vi "Test2_3a_ASIC_mezzanine.vi"(4 "Voltages comprobation":dbl[](array[numeric])=[0.05, 0.1, 0.2, 0.3, 0.4, 0.5, 0.6, 0.7, 0.8, 1.0], 6 "IB_Clip":i32[](array[numeric])=[0, 1, 2, 3, 4, 5, 6], 7 "Report Enable":bool, 8 "error in":errorcluster, 9 "Cycles Burst":i32=10000, 10 "Channels":i32[](array[numeric])=[0, 1, 2, 3, 4, 5, 6], 11 "Instrument VISA in":T1={"AWG VISA"="generadorpulsos", "Oscilloscope  VISA "="Oscilloscope", "Integration Board IP"="172.16.7.43", "connection ID"=refnum, "report out"=refnum, "report file path"=path "D:/CTA/Data_test/ASIC/chip_test"}) -> (0 "error out":errorcluster, 3 "Instrument VISA out":T1={"AWG VISA"="generadorpulsos", "Oscilloscope  VISA "="Oscilloscope", "Integration Board IP"="172.16.7.43", "connection ID"=refnum, "report out"=refnum, "report file path"=path "D:/CTA/Data_test/test3a"})   [LabVIEW 2009]
uses:
  <vilib>/Utility/NIReport.llb/NI_report.lvclass
  <vilib>/Utility/NIReport.llb/HTML/NI_HTML.lvclass
  <instrlib>/Agilent 8000 Series/Public/Configure/Configure Math (Binary Operation).vi
  <instrlib>/Agilent 8000 Series/Public/Data/Read (Multiple Waveforms).vi
  L0 Asic Test Folder v9/C/Program Files/National Instruments/LabVIEW 2012/instr.lib/Agilent 81150/Agilent 81150.lvlib
  L0 Asic Test Folder v9/C/Program Files/National Instruments/LabVIEW 2012/instr.lib/Agilent 8000 Series/Agilent 8000 Series.lvlib
panel:
  in  "Atenuation":i32[](array[numeric])=[0, 4, 8, 12]
  in  "Generador enable?":bool=TRUE
  out "dt":dbl
  out "report file path":path=path "D:/CTA/Data_test/ASIC/chip_test"
  in  "Full waveform":bool
  out "Waveform Data":waveform(dbl)[](graph)
  out "x-y 4":u32=42918
  in  "y":dbl=250.0
  out "bucle":u16
  out "x-y 3":u32=42918
  out "points quantity":dbl=104.0
  out "appended array":dbl[](array[numeric])=[1.222, 0.0079, 2.4586e-09, 6.8e-12, 0.009395, 0.004623, 9.99999e+37, 9.99999e+37, 5.8615e-09, 1.47682e-09, 104.0]
  out "read buffer 3":string="V amptd(1),1.233E+00,0,1.206E+00,1.250E+00,1.2220E+00,7.9E-03,1.04E+02,+ width(f1),2.471E-09,1,2.449E-09,2.472E-09,2.4586E-09,6.8E-12,1.03E+02,V amptd(f2),8.62E-03,1,1.99E-03,3.271E-02,9.395E-03,4.623E-03,1.04E+02,+ width(f2),9.99999E+37,5,9.99999E+37,9.99999E+37,9.99999E+37,9.99999E+37,9.99999E+37,Time(f1-f2),9.99999E+37,5,4.91554E-09,8.06319E-09,5.86150E-09,1.47682E-09,4E+00\n"
  out "x-y":u32=956
  out "Numeric":i32=2147483647
  in  "Att gain":u32=4095
  in  "Save NOW!":bool
  in  "End 2":bool=TRUE
  out "Data output":dbl[][](array[numeric])
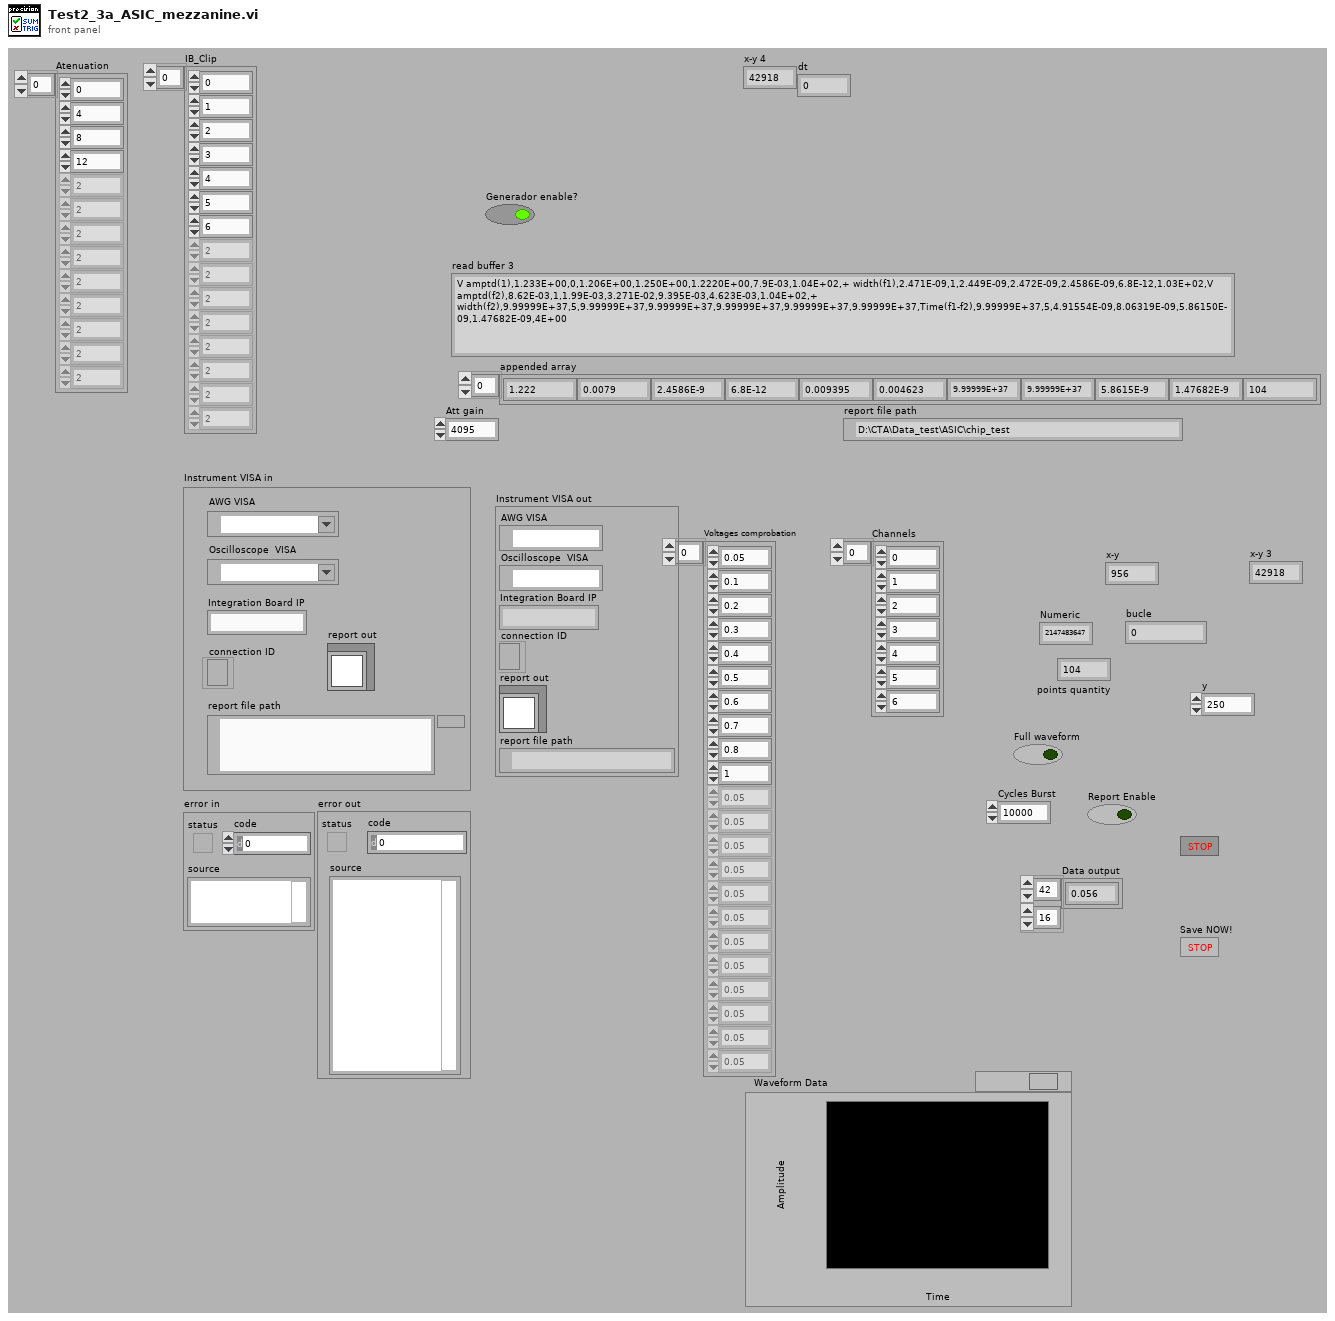
[diagram p1: front panel]
types:
  T1 = cluster{"AWG VISA":refnum<visa-resource-name>, "Oscilloscope  VISA ":refnum<visa-resource-name>, "Integration Board IP":string, "connection ID":refnum<k5>, "report out":refnum<class "NI_report.lvclass">, "report file path":path}
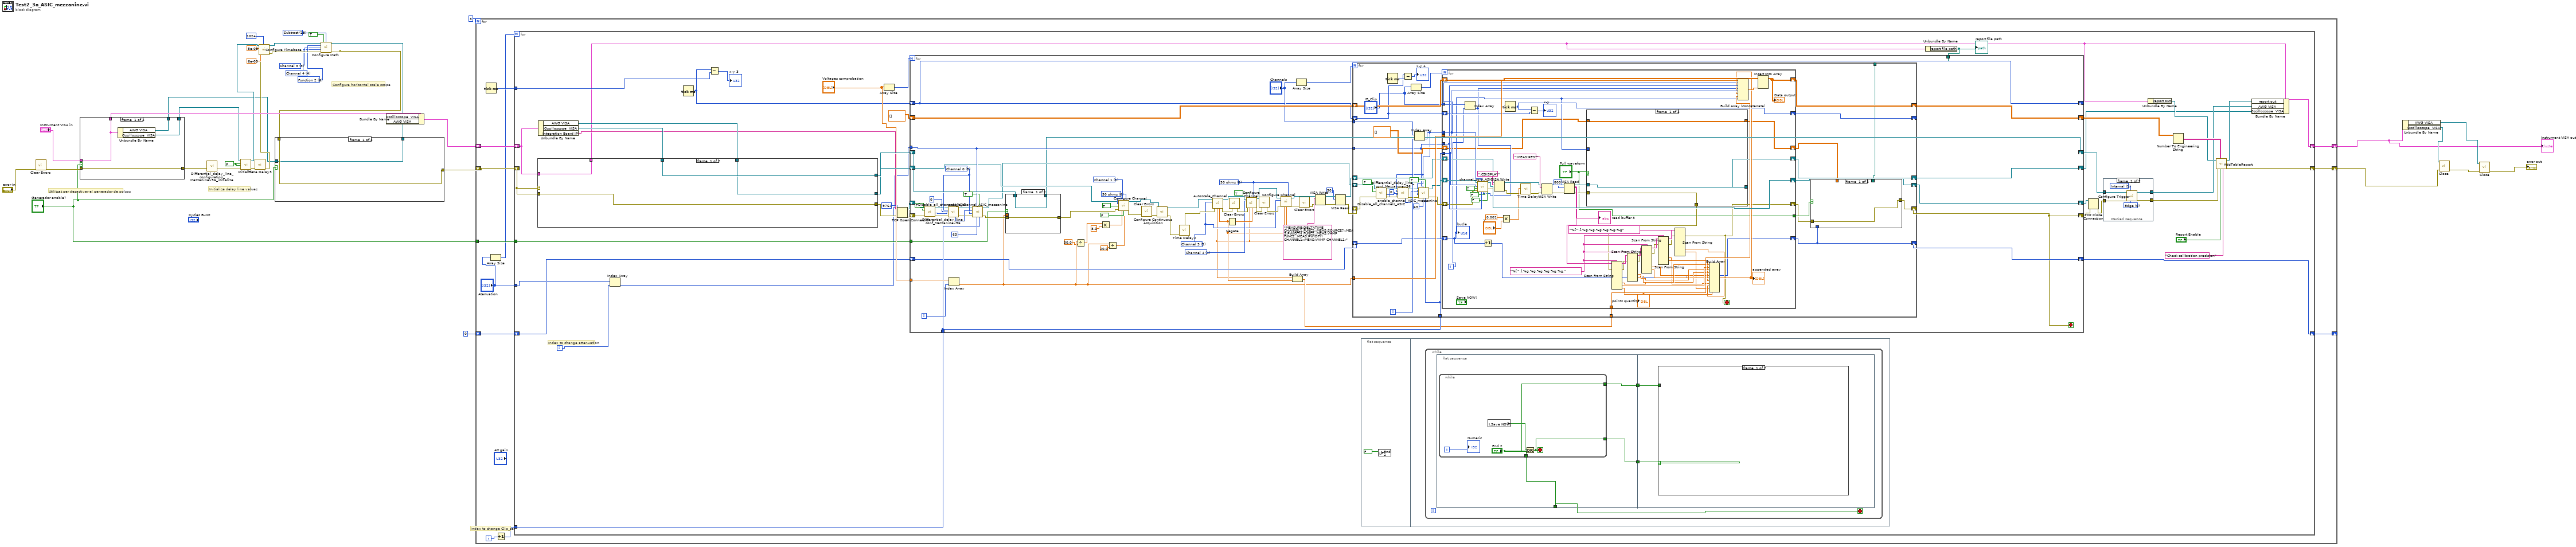
[diagram p0: block diagram]
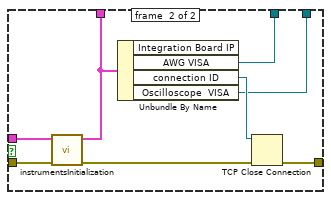
[diagram p2: hidden frame]
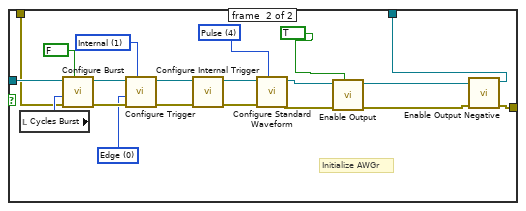
[diagram p3: hidden frame]
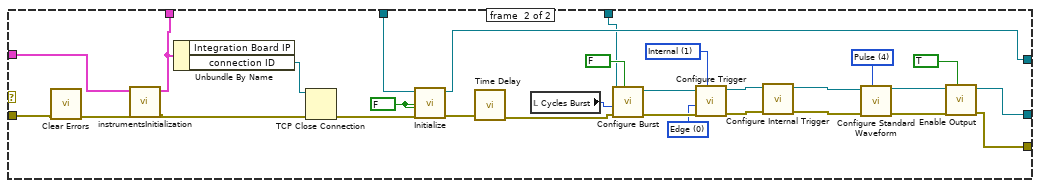
[diagram p4: hidden frame]
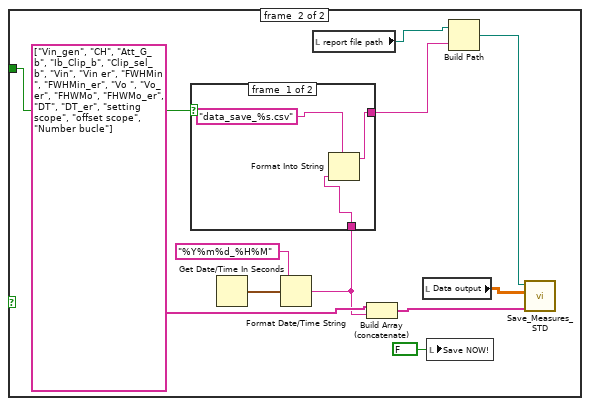
[diagram p5: hidden frame]
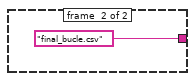
[diagram p6: hidden frame]
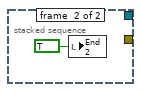
[diagram p7: hidden frame]
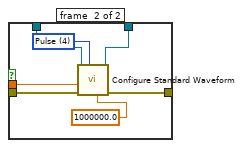
[diagram p8: hidden frame]
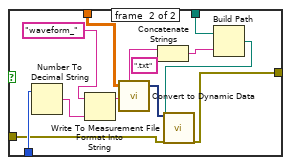
[diagram p9: hidden frame]
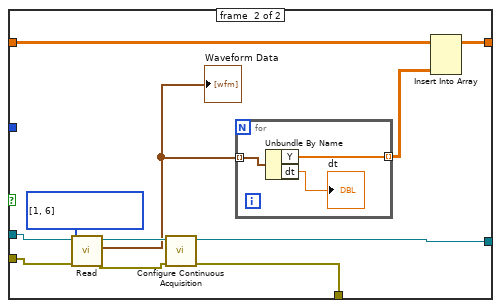
[diagram p10: hidden frame]
diagram:
  w24 = u16 6 items=["Function 1"=5, "Function 2"=6, "Function 3"=7, "Function 4"=8] ("Math Channel (5: Function 1)")
  w28 = u16 15 items=["Add"=12, "Divide"=13, "Multiply"=14, "Subtract"=15, "Common Mode"=16, "Versus"=17] ("Math Operation (12: Add)")
  w23 = 3 items=["Channel 1"=1, "Channel 2"=2, "Channel 3"=3, "Channel 4"=4] ("Channel (1: Channel 1)")
  w22 = 4 items=["Channel 1"=1, "Channel 2"=2, "Channel 3"=3, "Channel 4"=4] ("Channel (1: Channel 1)")
  w36 = FALSE ("ID Query (True)")
  # "Configure horizontal scale scope"
  # "Initialize delay line values"
  # "Utilitzat per desactivar el generador de polsos"
  # "Index to change Clip_sel"
  n1 = call <vilib>:"Clear Errors.vi"("error in (no error)"="error in") -> ("error out"=w34:errorcluster)  [unwired: 6 in]
  n2 = case shown="True" "Generador enable?" {
    tunnel: w34 -> [w40 w48]
    tunnel: "Instrument VISA in" -> [w37 w47]
    tunnel: [w37 w46] -> w31
    tunnel: [w40 w41] -> w4
    tunnel: [w39 w43] -> w3
    tunnel: [w38 w44] -> w2
    frame #0 {
      n3 = Unbundle By Name(w37) -> ("AWG VISA"=w39:refnum<visa-resource-name>, "Oscilloscope  VISA"=w38:refnum<visa-resource-name>)
    }
    frame #1 {
      n4 = call "instrumentsInitialization.vi"("error in"=w48, "Instrument VISA in"=w47) -> ("error out"=w42:errorcluster, "Instrument VISA out"=w46:T1)  [unwired: 8 in]
      n5 = Unbundle By Name(w46) -> ("AWG VISA"=w43:refnum<visa-resource-name>, "connection ID"=w45:refnum<k5>, "Oscilloscope  VISA"=w44:refnum<visa-resource-name>)  [unwired: 1 out]
      n6 = TCP Close Connection(connection ID=w45, error in (no error)=w42) -> (error out=w41:errorcluster)  [unwired: 1 in, 1 out]
    }
  }
  n7 = call "Differential_delay_line_configuration_Mezzaninev56_initialize.vi"("error in (no error)"=w4) -> ("error out 2"=w5:errorcluster)  [unwired: 1 in]
  n8 = call "Initialize.vi"("error in (no error)"=w5, "Reset (True)"=w36, "ID Query (True)"=w36, "VISA resource name"=w2) -> ("error out"=w35:errorcluster, "VISA resource name out"=w21:refnum<visa-resource-name>)  [unwired: 6 in]
  n9 = call "Time Delay3"("error in (no error)"=w35) -> ("error out"=w20:errorcluster)  [unwired: 10 in]
  n10 = call "Configure Timebase.vi"("Record Length (1000)"=1024, "error in (no error)"=w20, "Position (0.0 s)"=6e-09, "Timebase (0.005 s)"=5e-08, "VISA resource name"=w21) -> ("error out"=w25:errorcluster, "VISA resource name out"=w26:refnum<visa-resource-name>)  [unwired: 5 in]
  n11 = call-poly <instrlib>:"Configure Math.vi"("VISA resource name"=w26, "Enable Math Channel (T:Enable)"=TRUE, "Math Operation (12: Add)"=w28, "Math Channel (5: Function 1)"=w24, "Math Operand (1: Channel 1)"=w23, "Math Operand (2: Channel 2)"=w22, "error in (no error)"=w25) -> ("VISA resource name out"=w9:refnum<visa-resource-name>, "error out"=w10:errorcluster)  [unwired: 7 in]
  n12 = case shown="True" "Generador enable?" {
    tunnel: w3 -> [w49 w59]
    tunnel: w10 -> [w50 w55]
    tunnel: [w50 w53] -> w7
    tunnel: [w49 w51] -> w6
    frame #0 {
    }
    frame #1 {
      w64 = u16 1 items=["Immediate", "Internal", "External", "Software Trigger Function"] ("Trigger Source (0: Immediate)")
      w65 = u16 0 items=["Edge", "Level"] ("Trigger Mode (0: Edge)")
      w69 = u16 4 items=["Sine", "Square", "Ramp Up", "Ramp Down", "Pulse", "Noise", "DC"] ("Waveform (0: Sine)")
      # "Initialize AWGr"
      n13 = local read "Cycles Burst"() -> (w68:i32)
      n14 = call "Configure Burst.vi"("Enable Burst (F: Disable)"=FALSE, "error in (no error)"=w55, "Burst Count (2)"=w68, "VISA resource name"=w59) -> ("error out"=w67:errorcluster, "VISA resource name out"=w66:refnum<visa-resource-name>)  [unwired: 6 in]
      n15 = call "Configure Trigger.vi"("Trigger Source (0: Immediate)"=w64, "error in (no error)"=w67, "Trigger Mode (0: Edge)"=w65, "VISA resource name"=w66) -> ("error out"=w63:errorcluster, "VISA resource name out"=w62:refnum<visa-resource-name>)  [unwired: 6 in]
      n16 = call "Configure Internal Trigger.vi"("error in (no error)"=w63, "VISA resource name"=w62) -> ("error out"=w60:errorcluster, "VISA resource name out"=w61:refnum<visa-resource-name>)  [unwired: 8 in]
      n17 = call "Configure Standard Waveform.vi"("Waveform (0: Sine)"=w69, "error in (no error)"=w60, "VISA resource name"=w61) -> ("error out"=w58:errorcluster, "VISA resource name out"=w57:refnum<visa-resource-name>)  [unwired: 7 in]
      n18 = call "Enable Output.vi"("Enable Output (T: Enable)"=TRUE, "error in (no error)"=w58, "VISA resource name"=w57) -> ("error out"=w54:errorcluster, "VISA resource name out"=w52:refnum<visa-resource-name>)  [unwired: 7 in]
      n19 = call "Enable Output Negative.vi"("error in (no error)"=w54, "VISA resource name"=w52) -> ("error out"=w53:errorcluster, "VISA resource name out"=w51:refnum<visa-resource-name>)  [unwired: 8 in]
    }
  }
  n20 = Bundle By Name(cluster=w31, "Oscilloscope  VISA"=w9, "AWG VISA"=w6) -> (w12:T1)
  n21 = for {
    N: 3 -> [_]
    shift-right: [w82] -> w15
    shift-left: w7 -> [w78]
    shift-right: [w81] -> w13
    shift-left: w12 -> [w77]
    shift-right: [w74] -> _
    shift-left: u16 0 ("remote port or service name") -> [w75]
    tunnel: "Generador enable?" -> [w73]
    i -> [w79]
    n22 = Tick Count (ms)() -> (millisecond timer value=w76:u32)
    n23 = Array Size(array="Atenuation") -> (size(s)=w71:i32)
    n24 = Increment(x=w79) -> (x+1=w80:i32)
    n25 = for {
      N: w71 -> [_]
      shift-right: [w114] -> w82
      shift-left: w78 -> [w108]
      shift-right: [w112] -> w81
      shift-left: w77 -> [w113]
      tunnel: w80 -> [w87]
      tunnel: w76 -> [w94]
      shift-right: [w92] -> w74
      shift-left: w75 -> [w93]
      tunnel: w73 -> [w86]
      tunnel: "Atenuation" -> [w84]
      i -> [w83]
      # "Index to change attenuation"
      n26 = Unbundle By Name(w113) -> ("AWG VISA"=w107:refnum<visa-resource-name>, "Oscilloscope  VISA"=w110:refnum<visa-resource-name>, "Integration Board IP"=w103:string)
      n27 = case shown="Error" w108 {
        tunnel: w113 -> [w127 w156]
        tunnel: w108 -> [w126 w150]
        tunnel: [w127 w155] -> w89
        tunnel: [w126 w132] -> w102
        tunnel: w110 -> [w125 w154]
        tunnel: [w125 w153] -> w109
        tunnel: w107 -> [w124 w134]
        tunnel: [w124 w133] -> w106
        frame #0 {
        }
        frame #1 {
          w139 = u16 1 items=["Immediate", "Internal", "External", "Software Trigger Function"] ("Trigger Source (0: Immediate)")
          w140 = u16 0 items=["Edge", "Level"] ("Trigger Mode (0: Edge)")
          w147 = u16 4 items=["Sine", "Square", "Ramp Up", "Ramp Down", "Pulse", "Noise", "DC"] ("Waveform (0: Sine)")
          w152 = FALSE ("ID Query (True)")
          n28 = call <vilib>:"Clear Errors.vi"("error in (no error)"=w150) -> ("error out"=w149:errorcluster)  [unwired: 6 in]
          n29 = call "instrumentsInitialization.vi"("error in"=w149, "Instrument VISA in"=w156) -> ("error out"=w129:errorcluster, "Instrument VISA out"=w155:T1)  [unwired: 8 in]
          n30 = Unbundle By Name(w155) -> ("connection ID"=w130:refnum<k5>)  [unwired: 1 out]
          n31 = TCP Close Connection(connection ID=w130, error in (no error)=w129) -> (error out=w128:errorcluster)  [unwired: 1 in, 1 out]
          n32 = call "Initialize.vi"("error in (no error)"=w128, "Reset (True)"=w152, "ID Query (True)"=w152, "VISA resource name"=w154) -> ("error out"=w151:errorcluster, "VISA resource name out"=w153:refnum<visa-resource-name>)  [unwired: 6 in]
          n33 = call "Time Delay"("error in (no error)"=w151) -> ("error out"=w131:errorcluster)  [unwired: 10 in]
          n34 = local read "Cycles Burst"() -> (w143:i32)
          n35 = call "Configure Burst.vi"("Enable Burst (F: Disable)"=FALSE, "error in (no error)"=w131, "Burst Count (2)"=w143, "VISA resource name"=w134) -> ("error out"=w142:errorcluster, "VISA resource name out"=w141:refnum<visa-resource-name>)  [unwired: 6 in]
          n36 = call "Configure Trigger.vi"("Trigger Source (0: Immediate)"=w139, "error in (no error)"=w142, "Trigger Mode (0: Edge)"=w140, "VISA resource name"=w141) -> ("error out"=w138:errorcluster, "VISA resource name out"=w137:refnum<visa-resource-name>)  [unwired: 6 in]
          n37 = call "Configure Internal Trigger.vi"("error in (no error)"=w138, "VISA resource name"=w137) -> ("error out"=w135:errorcluster, "VISA resource name out"=w136:refnum<visa-resource-name>)  [unwired: 8 in]
          n38 = call "Configure Standard Waveform.vi"("Waveform (0: Sine)"=w147, "error in (no error)"=w135, "VISA resource name"=w136) -> ("error out"=w146:errorcluster, "VISA resource name out"=w145:refnum<visa-resource-name>)  [unwired: 7 in]
          n39 = call "Enable Output.vi"("Enable Output (T: Enable)"=TRUE, "error in (no error)"=w146, "VISA resource name"=w145) -> ("error out"=w132:errorcluster, "VISA resource name out"=w133:refnum<visa-resource-name>)  [unwired: 7 in]
        }
      }
      n40 = Index Array(array=w84, index=w83) -> (element=w85:i32)
      n41 = Tick Count (ms)() -> (millisecond timer value=w95:u32)
      n42 = Subtract(x=w95, y=w94) -> (x-y=→"x-y 3":u32)
      n43 = Array Size(array="Voltages comprobation") -> (size(s)=w115:i32)
      n44 = TCP Open Connection(address=w103, remote port or service name=u16 9764, error in (no error)=w102) -> (connection ID=w97:refnum<k5>, error out=w101:errorcluster)  [unwired: 2 in]
      n45 = flat-sequence {
        frame #0 {
          n46 = local write "End 2"(FALSE ("End")) -> ()
        }
        frame #1 {
          n47 = while {
            stop <- w158 stop-if-true
            n48 = flat-sequence {
              tunnel: [w163] -> w160
              tunnel: [w162] -> w159
              tunnel: [w161] -> w158
              tunnel: w160 -> [w169]
              tunnel: w159 -> [w168]
              frame #0 {
                n49 = while {
                  tunnel: [w166] -> w163
                  tunnel: ["End 2"] -> w162
                  tunnel: ["End 2"] -> w161
                  i -> [w165]
                  stop <- w166 stop-if-true
                  n50 = local read "Save NOW!"() -> (w167:bool)
                  n51 = Or(x=w167, y="End 2") -> (x .or. y?=w166:bool)
                  "Numeric" <- w165
                }
              }
              frame #1 {
                n52 = case shown="True" w169 {
                  tunnel: w168 -> [_ w177]
                  frame #0 {
                  }
                  frame #1 {
                    n53 = Get Date/Time In Seconds() -> (seconds since 1Jan1904=w173:timestamp)
                    n54 = Format Date/Time String(time format string (%c)="%Y%m%d_%H%M", seconds (now)=w173) -> (date/time string=w171:string)  [unwired: 1 in]
                    n55 = case shown="False" w177 {
                      tunnel: [w182 "final_bucle.csv" ("format string")] -> w176
                      tunnel: w171 -> [w181 _]
                      frame #0 {
                        n56 = Format Into String(format string="data_save_%s.csv", w181) -> (resulting string=w182:string)  [unwired: 2 in, 1 out]
                      }
                      frame #1 {
                      }
                    }
                    n57 = local read "report file path"() -> (w170:path)
                    n58 = Build Array (concatenate)(string[] ["Vin_gen", "CH", "Att_G_b", "Ib_Clip_b", "Clip_sel_b", "Vin", "Vin er", "FWHMin ", "FWHMin_er", "Vo ", "Vo_er", "FHWMo", "FHWMo_er", "DT", "DT_er", "setting scope", "offset scope", "Number bucle"] ("appended array"), w171) -> (w174:string[])
                    n59 = local read "Data output"() -> (w179:dbl[][])
                    n60 = local write "Save NOW!"(FALSE ("Save NOW!")) -> ()
                    n61 = Build Path(base path=w170, name or relative path=w176) -> (appended path=w180:path)
                    n62 = call "Save_Measures_STD.vi"("appended array"=w174, "Data in"=w179, "file path (dialog if empty)"=w180) -> ()  [unwired: 9 in]
                  }
                }
              }
            }
          }
        }
      }
      n63 = Unbundle By Name(w89) -> ("report file path"=w88:path)
      "report file path" <- w88
      n64 = for {
        N: w115 -> [_]
        shift-right: [w204] -> w99
        shift-left: w101 -> [w236]
        shift-right: [w259] -> w119
        shift-left: dbl[][] [] -> [w260]
        tunnel: "Voltages comprobation" -> [w258]
        shift-right: [w224] -> w111
        shift-left: w106 -> [w266]
        shift-right: [w252] -> w90
        shift-left: w109 -> [w241]
        tunnel: w85 -> [w250]
        tunnel: w87 -> [w247]
        shift-right: [w235] -> w98
        shift-left: w97 -> [w234]
        shift-right: [w207] -> _
        shift-left: w95 -> [w207]
        shift-right: [w206] -> w92
        shift-left: w93 -> [w220]
        tunnel: w88 -> [w205]
        tunnel: w86 -> [w192]
        i -> [w265]
        stop <- w204 stop-if-true
        w213 = 3 items=["Channel 1"=1, "Channel 2"=2, "Channel 3"=3, "Channel 4"=4] ("Channel (1: Channel 1)")
        w237 = 4 items=["Channel 1"=1, "Channel 2"=2, "Channel 3"=3, "Channel 4"=4] ("Channel (1: Channel 1)")
        w214 = u32 0 items=["50 ohms", "1 Mohms"] ("Input Impedance (1: 1 Mohms)")
        w199 = u16 0 items=["Channel 0", "Channel 1", "Channel 2", "Channel 3", "Channel 4", "Channel 5", "Channel 6"] ("Channel")
        w262 = u32 0 items=["50 ohms", "1 Mohms"] ("Input Impedance (1: 1 Mohms)")
        w264 = 1 items=["Channel 1"=1, "Channel 2"=2, "Channel 3"=3, "Channel 4"=4] ("Channel (1: Channel 1)")
        n65 = call "Disable_all_channels_ASIC.vi"("error in"=w236, "Clip_en_b"=FALSE, "connection ID"=w234) -> ("error out"=w200:errorcluster, "id_out"=w203:i32, "connection ID out"=w197:refnum<k5>)  [unwired: 6 in]
        n66 = call "Differential_delay_line_conf_Mezzaninev56.vi"("connection ID"=w197, "channel"=w199, "Delay value"=u16 0, "Id in"=w203, "error in (no error)"=w200) -> ("connection ID out"=w198:refnum<k5>, "Id out"=w202:i32, "error out 2"=w201:errorcluster)  [unwired: 3 in, 5 out]
        n67 = Index Array(array=w258, index=w265) -> (element=w195:dbl)
        n68 = call "enable_channel_ASIC_mezzanine.vi"("Clip_sel_b"=w247, "maj/sum"=TRUE, "Ib_clipVb"=u32 63, "Att gain"=w250, "error in"=w201, "Channel"=w199, "id_in"=w202, "connection ID"=w198) -> ("error out"=w251:errorcluster, "connection ID out"=w226:refnum<k5>)  [unwired: 1 in, 1 out]
        n69 = case shown="True" w192 {
          tunnel: w266 -> [w267 w273]
          tunnel: w251 -> [w268 w272]
          tunnel: [w268 w271] -> w242
          tunnel: [w267 w270] -> w224
          tunnel: w195 -> [_ w269]
          frame #0 {
          }
          frame #1 {
            w274 = u16 4 items=["Sine", "Square", "Ramp Up", "Ramp Down", "Pulse", "Noise", "DC"] ("Waveform (0: Sine)")
            n70 = call "Configure Standard Waveform.vi"("Frequency (1000.0 Hz)"=1000000.0, "Waveform (0: Sine)"=w274, "error in (no error)"=w272, "Amplitude (1.0 Vpp)"=w269, "VISA resource name"=w273) -> ("error out"=w271:errorcluster, "VISA resource name out"=w270:refnum<visa-resource-name>)  [unwired: 5 in]
          }
        }
        n71 = Divide(x=w195, y=30.0) -> (x/y=w193:dbl)
        n72 = Multiply(x=w193, y=8.0) -> (x*y=w245:dbl)
        n73 = Divide(x=w195, y=20.0) -> (x/y=w249:dbl)
        n74 = call "Configure Channel.vi"("VISA resource name"=w241, "Enable Channel (Enable)"=TRUE, "BW Limit 20MHz (Disable)"=FALSE, "Input Impedance (1: 1 Mohms)"=w262, "Channel (1: Channel 1)"=w264, "error in (no error)"=w242, "Vertical Range (2.0 V)"=w245, "Vertical Offset (0.0 V)"=w249) -> ("VISA resource name out"=w240:refnum<visa-resource-name>, "error out"=w239:errorcluster)  [unwired: 6 in]
        n75 = call <vilib>:"Clear Errors.vi"("error in (no error)"=w239) -> ("error out"=w238:errorcluster)  [unwired: 6 in]
        n76 = call "Configure Continuous Acquisition.vi"("error in (no error)"=w238, "VISA resource name"=w240) -> ("error out"=w248:errorcluster, "VISA resource name out"=w232:refnum<visa-resource-name>)  [unwired: 8 in]
        n77 = call "Time Delay2"("error in (no error)"=w248) -> ("error out"=w233:errorcluster)  [unwired: 10 in]
        n78 = call "Autoscale_Channel.vi"("error in"=w233, "Channel"=w213, "VISA resource name"=w232) -> ("error out"=w253:errorcluster, "VISA resource name out"=w256:refnum<visa-resource-name>, "Offset"=w212:dbl, "VerticalRange"=w211:dbl)  [unwired: 5 in]
        n79 = Negate(x=w212) -> (-x=w243:dbl)
        n80 = call <vilib>:"Clear Errors.vi"("error in (no error)"=w253) -> ("error out"=w254:errorcluster)  [unwired: 6 in]
        n81 = call "Configure Channel.vi"("VISA resource name"=w256, "Enable Channel (Enable)"=TRUE, "Input Impedance (1: 1 Mohms)"=w214, "Channel (1: Channel 1)"=w237, "error in (no error)"=w254, "Vertical Range (2.0 V)"=w211, "Vertical Offset (0.0 V)"=w243) -> ("VISA resource name out"=w216:refnum<visa-resource-name>, "error out"=w255:errorcluster)  [unwired: 7 in]
        n82 = call <vilib>:"Clear Errors.vi"("error in (no error)"=w255) -> ("error out"=w218:errorcluster)  [unwired: 6 in]
        n83 = call "Configure Channel.vi"("VISA resource name"=w216, "Input Impedance (1: 1 Mohms)"=w214, "Channel (1: Channel 1)"=w213, "error in (no error)"=w218, "Vertical Range (2.0 V)"=w211, "Vertical Offset (0.0 V)"=w212) -> ("VISA resource name out"=w215:refnum<visa-resource-name>, "error out"=w219:errorcluster)  [unwired: 8 in]
        n84 = Build Array(w211, w212) -> (w244:dbl[])
        n85 = Array Size(array="Channels") -> (size(s)=w225:i32)
        n86 = call <vilib>:"Clear Errors.vi"("error in (no error)"=w219) -> ("error out"=w217:errorcluster)  [unwired: 6 in]
        n87 = VISA Write(VISA resource name=w215, write buffer="MEASURE:DELTATIME CHANNEL1,FUNC2;:MEAS:SOURCE?;:MEAS:PWIDTH FUNC2;:MEAS:VAMP FUNC2;:MEAS:PWIDTH CHANNEL1;:MEAS:VAMP CHANNEL1;", error in (no error)=w217) -> (VISA resource name out=w231:refnum<visa-resource-name>, error out=w230:errorcluster)  [unwired: 1 out]
        n88 = VISA Read(VISA resource name=w231, byte count=u32 50, error in (no error)=w230) -> (VISA resource name out=w227:refnum<visa-resource-name>, error out=w228:errorcluster)  [unwired: 2 out]
        n89 = for {
          N: w225 -> [_]
          tunnel: w250 -> [w278]
          tunnel: w247 -> [w299]
          tunnel: w195 -> [w312]
          tunnel: w244 -> [w311]
          shift-right: [w314] -> w259
          shift-left: w260 -> [w315]
          shift-right: [w313] -> w252
          shift-left: w227 -> [w309]
          shift-right: [w310] -> w235
          shift-left: w226 -> [w303]
          shift-right: [w291] -> w204
          shift-left: w228 -> [w305]
          tunnel: "Channels" -> [w308]
          shift-right: [w287] -> w206
          shift-left: w220 -> [w306]
          shift-right: [w293] -> _
          shift-left: w207 -> [w294]
          tunnel: w205 -> [w289]
          i -> [w307]
          n90 = call "Disable_all_channels_ASIC.vi"("error in"=w305, "Clip_en_b"=FALSE, "connection ID"=w303) -> ("error out"=w283:errorcluster, "id_out"=w279:i32, "connection ID out"=w285:refnum<k5>)  [unwired: 6 in]
          n91 = Tick Count (ms)() -> (millisecond timer value=w295:u32)
          n92 = Subtract(x=w294, y=w295) -> (x-y=→"x-y 4":u32)
          n93 = Array Size(array="IB_Clip") -> (size(s)=w297:i32)
          n94 = Index Array(array=w308, index=w307) -> (element=w277:i32)
          n95 = call "Differential_delay_line_conf_Mezzaninev56.vi"("connection ID"=w285, "channel"=w277, "Delay value"=u16 0, "Id in"=w279, "error in (no error)"=w283) -> ("connection ID out"=w284:refnum<k5>, "Id out"=w281:i32, "error out 2"=w282:errorcluster)  [unwired: 3 in, 5 out]
          n96 = call "enable_channel_ASIC_mezzanine.vi"("Clip_sel_b"=w299, "maj/sum"=TRUE, "Ib_clipVb"=u32 63, "Att gain"=w278, "error in"=w282, "Channel"=w277, "id_in"=w281, "connection ID"=w284) -> ("error out"=w304:errorcluster, "connection ID out"=w302:refnum<k5>)  [unwired: 1 in, 1 out]
          n97 = for {
            N: w297 -> [_]
            shift-right: [w332] -> w290
            shift-left: w304 -> [w359]
            tunnel: w312 -> [w394]
            shift-right: [w372] -> w314
            shift-left: w315 -> [w392]
            tunnel: w278 -> [w389]
            shift-right: [w335] -> w313
            shift-left: w309 -> [w361]
            tunnel: w299 -> [w388]
            shift-right: [w390] -> w310
            shift-left: w302 -> [w391]
            tunnel: w311 -> [w386]
            shift-right: [w384] -> w293
            shift-left: w294 -> [w385]
            tunnel: w277 -> [w342]
            shift-right: [w341] -> w287
            shift-left: w306 -> [w333]
            tunnel: "IB_Clip" -> [w340]
            shift-right: [w330] -> w288
            shift-left: dbl[][] [] ("Y") -> [w331]
            tunnel: ["Full waveform"] -> w292
            i -> [w339]
            stop <- w332 stop-if-true
            w354 = "%[^,],%g,%g,%g,%g,%g,%g," ("format string")
            n98 = Index Array(array=w340, index=w339) -> (element=w338:i32)
            n99 = call "channel_conf_ASIC.vi"("connection ID"=w391, "Ring"=w342, "Clip_sel_b"=w388, "CompBuf_en_b"=TRUE, "error out"=w359, "Att gain"=w389, "Ib_ClipVb"=w338, "Clip_en_b"=FALSE, "Att_en_b"=FALSE) -> ("connection ID out"=w390:refnum<k5>, "error out 2"=w357:errorcluster)  [unwired: 2 in, 3 out]
            n100 = Increment(x=w333) -> (x+1=w341:u16)
            n101 = VISA Write(VISA resource name=w361, write buffer=":CDISPLAY", error in (no error)=w357) -> (VISA resource name out=w363:refnum<visa-resource-name>, error out=w356:errorcluster)  [unwired: 1 out]
            n102 = Multiply(x=0.001, y="y") -> (x*y=w375:dbl)
            n103 = Tick Count (ms)() -> (millisecond timer value=w384:u32)
            n104 = call "Time Delay4"("error in (no error)"=w356, "Delay Time (s)"=w375) -> ("error out"=w374:errorcluster)  [unwired: 9 in]
            n105 = Subtract(x=w384, y=w385) -> (x-y=→"x-y":u32)
            n106 = VISA Write(VISA resource name=w363, write buffer=":MEAS:RES?", error in (no error)=w374) -> (VISA resource name out=w382:refnum<visa-resource-name>, error out=w381:errorcluster)  [unwired: 1 out]
            n107 = VISA Read(VISA resource name=w382, byte count=u32 800, error in (no error)=w381) -> (VISA resource name out=w336:refnum<visa-resource-name>, read buffer=w378:string, error out=w337:errorcluster)  [unwired: 1 out]
            "read buffer 3" <- w378
            n108 = case shown="True" "Full waveform" {
              tunnel: w337 -> [w397 w406]
              tunnel: w336 -> [w396 w408]
              tunnel: [w396 w404] -> w335
              tunnel: [w397 w398] -> w334
              tunnel: w333 -> [_ _]
              tunnel: w331 -> [w395 w401]
              tunnel: [w395 w400] -> w330
              frame #0 {
              }
              frame #1 {
                w407 = i32[] [1, 6] items=["Channel 1"=1, "Channel 2"=2, "Channel 3"=3, "Channel 4"=4, "Function 1"=5, "Function 2"=6, "Function 3"=7, "Function 4"=8, "Memory 1"=9, "Memory 2"=10, "Memory 3"=11, "Memory 4"=12] ("Channels")
                n109 = call-poly <instrlib>:"Read.vi"("error in (no error)"=w406, "Channels"=w407, "VISA resource name"=w408) -> ("error out"=w403:errorcluster, "Waveform Data"=w402:waveform(dbl)[], "VISA resource name out"=w405:refnum<visa-resource-name>)  [unwired: 6 in]
                "Waveform Data" <- w402
                n110 = call "Configure Continuous Acquisition.vi"("error in (no error)"=w403, "VISA resource name"=w405) -> ("error out"=w398:errorcluster, "VISA resource name out"=w404:refnum<visa-resource-name>)  [unwired: 8 in]
                n111 = for {
                  tunnel: w402 -> [w411] mode=indexing
                  tunnel: [w410] -> w399 mode=indexing
                  n112 = Unbundle By Name(w411) -> ("Y"=w410:dbl[], "dt"=→"dt":dbl)
                }
                n113 = Insert Into Array(array=w401, new element=w399) -> (w400:dbl[][])  [unwired: 2 in]
              }
            }
            n114 = Scan From String(format string=w354, input string=w378, error in=w334) -> (remaining string=w371:string, error out=w364:errorcluster, output 5=w353:dbl, output 6=w351:dbl, output 7=w352:dbl)  [unwired: 12 in, 1 out]
            "points quantity" <- w352
            n115 = Scan From String(format string=w354, input string=w371, error in=w364) -> (remaining string=w368:string, error out=w365:errorcluster, output 5=w350:dbl, output 6=w349:dbl)  [unwired: 13 in, 1 out]
            n116 = Scan From String(format string=w354, input string=w368, error in=w365) -> (remaining string=w369:string, error out=w366:errorcluster, output 5=w348:dbl, output 6=w347:dbl)  [unwired: 13 in, 1 out]
            n117 = Scan From String(format string=w354, input string=w369, error in=w366) -> (remaining string=w370:string, error out=w367:errorcluster, output 5=w346:dbl, output 6=w345:dbl)  [unwired: 13 in, 1 out]
            n118 = Scan From String(format string="%[^,],%g,%g,%g,%g,%g,%g", input string=w370, error in=w367) -> (error out=w332:errorcluster, output 5=w344:dbl, output 6=w343:dbl)  [unwired: 13 in, 2 out]
            n119 = Build Array(w353, w351, w350, w349, w348, w347, w346, w345, w344, w343, w352) -> (w373:dbl[])
            "appended array" <- w373
            n120 = Build Array (concatenate)(w394, w342, w389, w338, w388, w373, w386, w333) -> (w393:dbl[])
            n121 = Insert Into Array(array=w392, new element=w393) -> (w372:dbl[][])  [unwired: 2 in]
            "Data output" <- w372
            "bucle" <- w333
          }
          n122 = case shown="True" w292 {
            tunnel: w288 -> [_ w328]
            tunnel: w290 -> [w316 w317]
            tunnel: [w316 w326] -> w291
            tunnel: w289 -> [_ w319]
            tunnel: w287 -> [_ w318]
            frame #0 {
            }
            frame #1 {
              n123 = Number To Decimal String(number=w318) -> (decimal integer string=w325:string)  [unwired: 1 in]
              n124 = Format Into String(initial string="waveform_", w325) -> (resulting string=w323:string)  [unwired: 2 in, 1 out]
              n125 = call "Convert to Dynamic Data"("2D Array"=w328) -> ("Dynamic Data Type"=w327:dynamicdata)  [unwired: 3 in]
              n126 = Concatenate Strings(w323, ".txt" ("string")) -> (w322:string)
              n127 = Build Path(base path=w319, name or relative path=w322) -> (appended path=w320:path)
              n128 = call "Write To Measurement File"("Signals"=w327, "error in (no error)"=w317, "Filename"=w320) -> ("error out"=w326:errorcluster)  [unwired: 14 in, 2 out]
            }
          }
        }
      }
      n129 = TCP Close Connection(connection ID=w98, error in (no error)=w99) -> (error out=w100:errorcluster)  [unwired: 1 in, 1 out]
      n130 = stacked-sequence {
        tunnel: w100 -> [w188 _]
        tunnel: [w187 _] -> w120
        tunnel: w111 -> [w186 _]
        tunnel: [w185 _] -> w91
        frame #0 {
          w189 = u16 1 items=["Immediate", "Internal", "External", "Software Trigger Function"] ("Trigger Source (0: Immediate)")
          w190 = u16 0 items=["Edge", "Level"] ("Trigger Mode (0: Edge)")
          n131 = call "Configure Trigger.vi"("Trigger Source (0: Immediate)"=w189, "error in (no error)"=w188, "Trigger Mode (0: Edge)"=w190, "VISA resource name"=w186) -> ("error out"=w187:errorcluster, "VISA resource name out"=w185:refnum<visa-resource-name>)  [unwired: 6 in]
        }
        frame #1 {
          n132 = local write "End 2"(TRUE ("End 2")) -> ()
        }
      }
      n133 = Unbundle By Name(w89) -> ("report out"=w116:refnum<class "NI_report.lvclass">)
      n134 = Number To Engineering String(4:w119) -> (0:w117:string[][])  [unwired: 3 in]
      n135 = call "AddTableReport.vi"("Table title"="Check calibration precision", "Report Enable"="Report Enable", "Data"=w117, "error in"=w120, "report in"=w116) -> ("error out"=w114:errorcluster, "report out"=w121:refnum<class "NI_report.lvclass">)  [unwired: 5 in]
      n136 = Bundle By Name(cluster=w89, "report out"=w121, "AWG VISA"=w91, "Oscilloscope  VISA"=w90) -> (w112:T1)
    }
  }
  "Instrument VISA out" <- w13
  n137 = Unbundle By Name(w13) -> ("AWG VISA"=w16:refnum<visa-resource-name>, "Oscilloscope  VISA"=w17:refnum<visa-resource-name>)
  n138 = call "Close.vi"("error in (no error)"=w15, "VISA resource name"=w17) -> ("error out"=w18:errorcluster)  [unwired: 9 in]
  n139 = call "Close.vi"("error in (no error)"=w18, "VISA resource name"=w16) -> ("error out"=→"error out":errorcluster)  [unwired: 9 in]
